vi "teste.vi"() -> ()   [LabVIEW 2019]
uses:
  <vilib>/Analysis/1siggen.llb/Ramp Pattern by Samples.vi
  <vilib>/Analysis/NI_AALBase.lvlib
panel:
  in  "frequencia":i32
  out "sinal":waveform(dbl)(graph)
  in  "amostras/s":i32
  in  "offset":dbl
  in  "amplitude":dbl
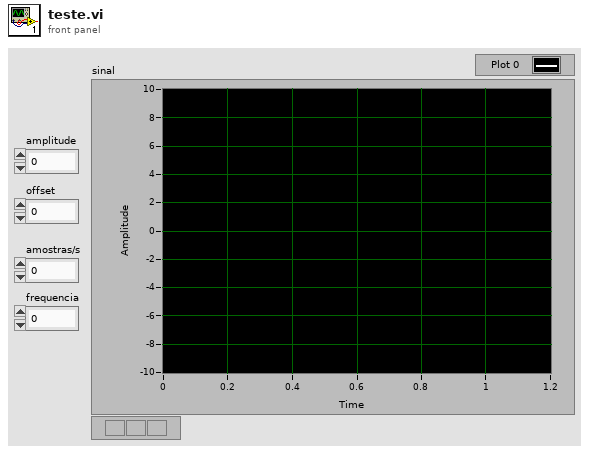
[diagram p1: front panel]
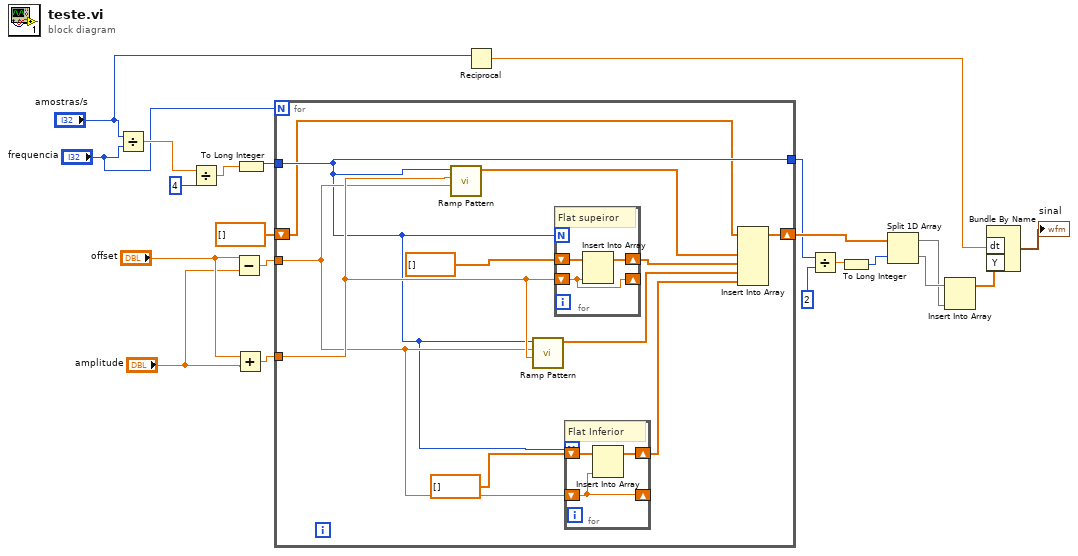
[diagram p0: block diagram]
diagram:
  n1 = Divide(x="amostras/s", y="frequencia") -> (x/y=w6:dbl)
  n2 = Divide(x=w6, y=4) -> (x/y=w16:dbl)
  n3 = Subtract(x="offset", y="amplitude") -> (x-y=w18:dbl)
  n4 = Add(x="offset", y="amplitude") -> (x+y=w19:dbl)
  n5 = To Long Integer(number=w16) -> (32bit integer=w13:i32)
  n6 = for {
    N: "frequencia" -> [_]
    tunnel: w19 -> [w30]
    tunnel: w18 -> [w29]
    tunnel: w13 -> [w23]
    tunnel: [w23] -> w8
    shift-right: [w24] -> w9
    shift-left: dbl[] [] -> [w22]
    n7 = call-poly <vilib>:"Ramp Pattern.vi"("start"=w29, "end"=w30, "samples"=w23) -> ("Ramp Pattern"=w28:dbl[])  [unwired: 7 in, 1 out]
    n8 = call-poly <vilib>:"Ramp Pattern.vi"("start"=w30, "end"=w29, "samples"=w23) -> ("Ramp Pattern"=w26:dbl[])  [unwired: 7 in, 1 out]
    n9 = for {
      N: w23 -> [_]
      shift-right: [w37] -> w27
      shift-left: dbl[] [] -> [w38]
      shift-right: [w36] -> _
      shift-left: w30 -> [w36]
      # "Flat supeiror"
      n10 = Insert Into Array(array=w38, new element=w36) -> (w37:dbl[])  [unwired: 1 in]
    }
    n11 = for {
      N: w23 -> [_]
      shift-right: [w34] -> w25
      shift-left: dbl[] [] -> [w35]
      shift-right: [w33] -> _
      shift-left: w29 -> [w33]
      # "Flat Inferior"
      n12 = Insert Into Array(array=w35, new element=w33) -> (w34:dbl[])  [unwired: 1 in]
    }
    n13 = Insert Into Array(array=w22, new element #1=w28, new element #2=w27, new element #3=w26, new element #4=w25) -> (w24:dbl[])  [unwired: 1 in]
  }
  n14 = Reciprocal(x="amostras/s") -> (1/x=w2:dbl)
  n15 = Divide(x=w8, y=2) -> (x/y=w15:dbl)
  n16 = To Long Integer(number=w15) -> (32bit integer=w14:i32)
  n17 = Split 1D Array(array=w9, index=w14) -> (first subarray=w10:dbl[], second subarray=w11:dbl[])
  n18 = Insert Into Array(array=w11, new element=w10) -> (w4:dbl[])  [unwired: 1 in]
  n19 = Bundle By Name("dt"=w2, "Y"=w4) -> (→"sinal":waveform(dbl))  [unwired: 1 in]
